vi "AC_2F2_ctl.vi"(8 "error in":errorcluster caption="错误输入（无错误）", 9 "Input2":T2, 11 "Input1":T3) -> (0 "error out":errorcluster caption="错误输出", 1 "AC2F2":T1={"自动请求状态"=FALSE, "空调按键引起弹窗显示"=FALSE, "最大制冷请求状态"=FALSE, "除霜请求状态"=FALSE, "内外循环进气"=0, "空气质量传感器请求"=FALSE, "吹风档位"=0, "负离子发生器状态"=0, "吹风模式"=0, "空调开启状态"=FALSE, "左侧设定温度"=18.0, "空调开关按键音"=FALSE, "AC远程控制模式与否"=FALSE, "空调按键触摸状态"=0, "空调按键状态"=0} {"空调按键状态" items=["No Press", "Blowup", "BlowDown", "AC Req", "MaxAcReq", "AUTOreq", "DefrostReq", "RearDefReq", "AirDistributionModeReq", "CycleReq", "DualReq", "IONreq", "AqsReq", "LeftTempUp", "LeftTempDown", "RightTempUp", "RightTempDown", "OFF", "KeyBLW"]; "空调按键触摸状态" items=["No Touch", "KeyLeftTemp", "KeyRightTemp", "KeyAUTO", "KeyAC", "KeyBLW+", "KeyBLW-", "KeyMODE", "KeyDEF", "KeyRearDEF", "KeyIntake", "KeyBLW", "Reserved"]; "左侧设定温度" min=17.5 max=31.5 step=0.5 scale=17.5..31.5 scale format="%#_6f"; "吹风模式" items=["Face", "Bilevel", "Foot", "FootScreen", "Screen", "预留", "无效"]; "负离子发生器状态" items=["关闭", "开启", "预留", "错误"]; "吹风档位" items=["关闭", "等级1", "等级2", "等级3", "等级4", "等级5", "等级6", "等级7", "等级8", "无效"]; "内外循环进气" items=["Fresh", "循环", "保持", "无效"]}, 3 "CmdStr":string)   [LabVIEW 2013]
uses:
  Input1.ctl
  Input2.ctl
  AC_2F2.ctl
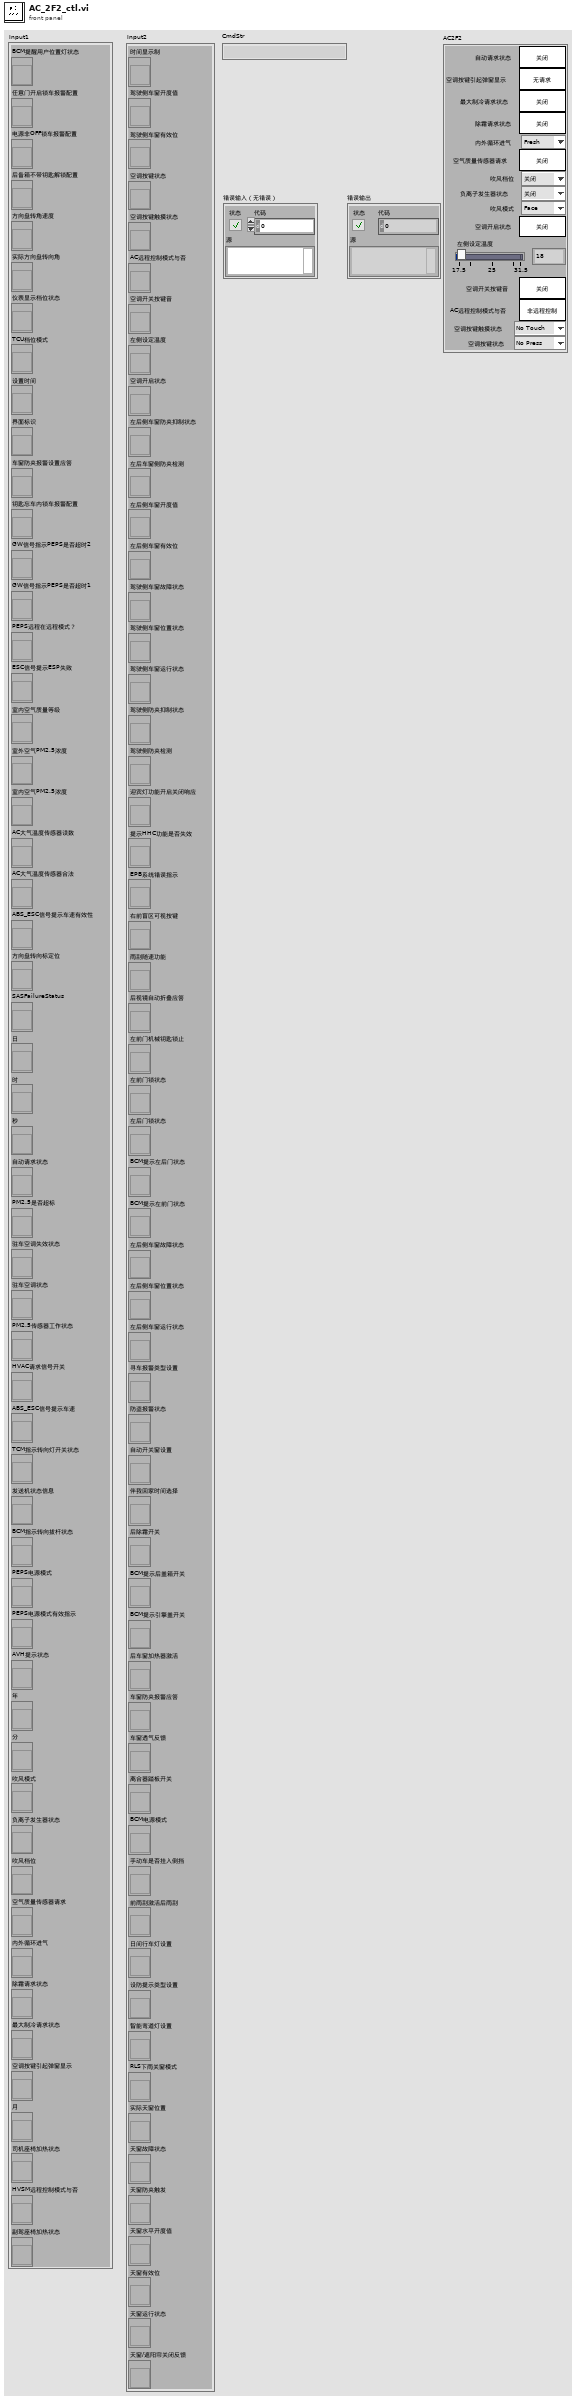
[diagram p1: front panel]
types:
  T1 = typedef "AC_2F2.ctl" = cluster{"自动请求状态":bool, "空调按键引起弹窗显示":bool, "最大制冷请求状态":bool, "除霜请求状态":bool, "内外循环进气":u16, "空气质量传感器请求":bool, "吹风档位":u16, "负离子发生器状态":u16, "吹风模式":u16, "空调开启状态":bool, "左侧设定温度":dbl, "空调开关按键音":bool, "AC远程控制模式与否":bool, "空调按键触摸状态":u16, "空调按键状态":u16}
  T2 = typedef "Input2.ctl" = cluster{"时间显示制":refnum<vi>, "驾驶侧车窗开度值":refnum<vi>, "驾驶侧车窗有效位":refnum<vi>, "空调按键状态":refnum<vi>, "空调按键触摸状态":refnum<vi>, "AC远程控制模式与否":refnum<vi>, "空调开关按键音":refnum<vi>, "左侧设定温度":refnum<vi>, "空调开启状态":refnum<vi>, "左后侧车窗防夹抑制状态":refnum<vi>, "左后车窗侧防夹检测":refnum<vi>, "左后侧车窗开度值":refnum<vi>, "左后侧车窗有效位":refnum<vi>, "驾驶侧车窗故障状态":refnum<vi>, "驾驶侧车窗位置状态":refnum<vi>, "驾驶侧车窗运行状态":refnum<vi>, "驾驶侧防夹抑制状态":refnum<vi>, "驾驶侧防夹检测":refnum<vi>, "迎宾灯功能开启关闭响应":refnum<vi>, "提示HHC功能是否失效":refnum<vi>, "EPB系统错误指示":refnum<vi>, "右前盲区可视按键":refnum<vi>, "雨刮随速功能":refnum<vi>, "后视镜自动折叠应答":refnum<vi>, "左前门机械钥匙锁止":refnum<vi>, "左前门锁状态":refnum<vi>, "左后门锁状态":refnum<vi>, "BCM提示左后门状态":refnum<vi>, "BCM提示左前门状态":refnum<vi>, "左后侧车窗故障状态":refnum<vi>, "左后侧车窗位置状态":refnum<vi>, "左后侧车窗运行状态":refnum<vi>, "寻车报警类型设置":refnum<vi>, "防盗报警状态":refnum<vi>, "自动开关窗设置":refnum<vi>, "伴我回家时间选择":refnum<vi>, "后除霜开关":refnum<vi>, "BCM提示后盖箱开关":refnum<vi>, "BCM提示引擎盖开关":refnum<vi>, "后车窗加热器激活":refnum<vi>, "车窗防夹报警应答":refnum<vi>, "车窗透气反馈":refnum<vi>, "离合器踏板开关":refnum<vi>, "BCM电源模式":refnum<vi>, "手动车是否挂入倒挡":refnum<vi>, "前雨刮激活后雨刮":refnum<vi>, "日间行车灯设置":refnum<vi>, "设防提示类型设置":refnum<vi>, "智能弯道灯设置":refnum<vi>, "RLS下雨关窗模式":refnum<vi>, "实际天窗位置":refnum<vi>, "天窗故障状态":refnum<vi>, "天窗防夹触发":refnum<vi>, "天窗水平开度值":refnum<vi>, "天窗有效位":refnum<vi>, "天窗运行状态":refnum<vi>, "天窗/遮阳帘关闭反馈":refnum<vi>}
  T3 = typedef "Input1.ctl" = cluster{"BCM提醒用户位置灯状态":refnum<vi>, "任意门开启锁车报警配置":refnum<vi>, "电源非OFF锁车报警配置":refnum<vi>, "后备箱不带钥匙解锁配置":refnum<vi>, "方向盘转角速度":refnum<vi>, "实际方向盘转向角":refnum<vi>, "仪表显示档位状态":refnum<vi>, "TCU档位模式":refnum<vi>, "设置时间":refnum<vi>, "界面标识":refnum<vi>, "车窗防夹报警设置应答":refnum<vi>, "钥匙忘车内锁车报警配置":refnum<vi>, "GW信号指示PEPS是否超时2":refnum<vi>, "GW信号指示PEPS是否超时1":refnum<vi>, "PEPS远程在远程模式？":refnum<vi>, "ESC信号提示ESP失败":refnum<vi>, "室内空气质量等级":refnum<vi>, "室外空气PM2.5浓度":refnum<vi>, "室内空气PM2.5浓度":refnum<vi>, "AC大气温度传感器读数":refnum<vi>, "AC大气温度传感器合法":refnum<vi>, "ABS_ESC信号提示车速有效性":refnum<vi>, "方向盘转向标定位":refnum<vi>, "SASFailureStatus":refnum<vi>, "日":refnum<vi>, "时":refnum<vi>, "秒":refnum<vi>, "自动请求状态":refnum<vi>, "PM2.5是否超标":refnum<vi>, "驻车空调失效状态":refnum<vi>, "驻车空调状态":refnum<vi>, "PM2.5传感器工作状态":refnum<vi>, "HVAC请求信号开关":refnum<vi>, "ABS_ESC信号提示车速":refnum<vi>, "TCM指示转向灯开关状态":refnum<vi>, "发送机状态信息":refnum<vi>, "BCM指示转向拔杆状态":refnum<vi>, "PEPS电源模式":refnum<vi>, "PEPS电源模式有效指示":refnum<vi>, "AVH提示状态":refnum<vi>, "年":refnum<vi>, "分":refnum<vi>, "吹风模式":refnum<vi>, "负离子发生器状态":refnum<vi>, "吹风档位":refnum<vi>, "空气质量传感器请求":refnum<vi>, "内外循环进气":refnum<vi>, "除霜请求状态":refnum<vi>, "最大制冷请求状态":refnum<vi>, "空调按键引起弹窗显示":refnum<vi>, "月":refnum<vi>, "司机座椅加热状态":refnum<vi>, "HVSM远程控制模式与否":refnum<vi>, "副驾座椅加热状态":refnum<vi>}
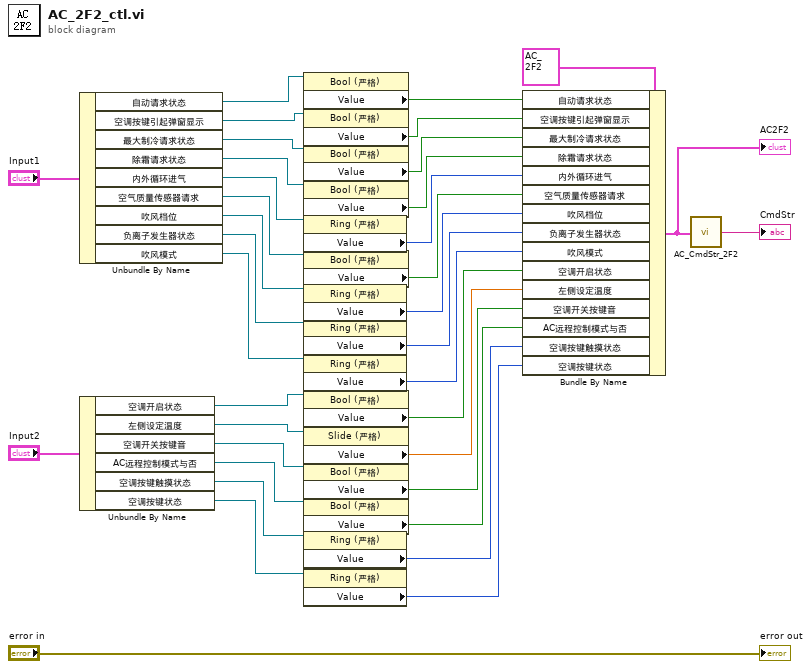
[diagram p0: block diagram]
diagram:
  n1 = Unbundle By Name("Input1") -> ("自动请求状态"=w32:refnum<vi>, "空调按键引起弹窗显示"=w30:refnum<vi>, "最大制冷请求状态"=w28:refnum<vi>, "除霜请求状态"=w26:refnum<vi>, "内外循环进气"=w24:refnum<vi>, "空气质量传感器请求"=w22:refnum<vi>, "吹风档位"=w20:refnum<vi>, "负离子发生器状态"=w18:refnum<vi>, "吹风模式"=w16:refnum<vi>)
  n2 = Unbundle By Name("Input2") -> ("空调开启状态"=w14:refnum<vi>, "左侧设定温度"=w12:refnum<vi>, "空调开关按键音"=w10:refnum<vi>, "AC远程控制模式与否"=w8:refnum<vi>, "空调按键触摸状态"=w6:refnum<vi>, "空调按键状态"=w4:refnum<vi>)
  n3 = property class="Bool (严格)"(reference=w32) -> ("Value"=w31:bool)  [unwired: 1 in, 2 out]
  n4 = property class="Bool (严格)"(reference=w30) -> ("Value"=w29:bool)  [unwired: 1 in, 2 out]
  n5 = property class="Bool (严格)"(reference=w28) -> ("Value"=w27:bool)  [unwired: 1 in, 2 out]
  n6 = property class="Bool (严格)"(reference=w26) -> ("Value"=w25:bool)  [unwired: 1 in, 2 out]
  n7 = property class="Ring (严格)"(reference=w24) -> ("Value"=w23:u16)  [unwired: 1 in, 2 out]
  n8 = property class="Bool (严格)"(reference=w22) -> ("Value"=w21:bool)  [unwired: 1 in, 2 out]
  n9 = property class="Ring (严格)"(reference=w20) -> ("Value"=w19:u16)  [unwired: 1 in, 2 out]
  n10 = property class="Ring (严格)"(reference=w18) -> ("Value"=w17:u16)  [unwired: 1 in, 2 out]
  n11 = property class="Ring (严格)"(reference=w16) -> ("Value"=w15:u16)  [unwired: 1 in, 2 out]
  n12 = property class="Bool (严格)"(reference=w14) -> ("Value"=w13:bool)  [unwired: 1 in, 2 out]
  n13 = property class="Slide (严格)"(reference=w12) -> ("Value"=w11:dbl)  [unwired: 1 in, 2 out]
  n14 = property class="Bool (严格)"(reference=w10) -> ("Value"=w9:bool)  [unwired: 1 in, 2 out]
  n15 = property class="Bool (严格)"(reference=w8) -> ("Value"=w7:bool)  [unwired: 1 in, 2 out]
  n16 = property class="Ring (严格)"(reference=w6) -> ("Value"=w5:u16)  [unwired: 1 in, 2 out]
  n17 = property class="Ring (严格)"(reference=w4) -> ("Value"=w3:u16)  [unwired: 1 in, 2 out]
  n18 = Bundle By Name(cluster=T1 {"自动请求状态"=FALSE, "空调按键引起弹窗显示"=FALSE, "最大制冷请求状态"=FALSE, "除霜请求状态"=FALSE, "内外循环进气"=0, "空气质量传感器请求"=FALSE, "吹风档位"=0, "负离子发生器状态"=0, "吹风模式"=0, "空调开启状态"=FALSE, "左侧设定温度"=18.0, "空调开关按键音"=FALSE, "AC远程控制模式与否"=FALSE, "空调按键触摸状态"=0, "空调按键状态"=0} ("AC命令输入"), "自动请求状态"=w31, "空调按键引起弹窗显示"=w29, "最大制冷请求状态"=w27, "除霜请求状态"=w25, "内外循环进气"=w23, "空气质量传感器请求"=w21, "吹风档位"=w19, "负离子发生器状态"=w17, "吹风模式"=w15, "空调开启状态"=w13, "左侧设定温度"=w11, "空调开关按键音"=w9, "AC远程控制模式与否"=w7, "空调按键触摸状态"=w5, "空调按键状态"=w3) -> (w33:T1)
  "AC2F2" <- w33
  n19 = call "AC_CmdStr_2F2.vi"("AC命令输入"=w33) -> ("CmdStr"=→"CmdStr":string)
  "error out" <- "error in"
